vi "NorthWest Window Control_Async.vi"(1 "Desired Window Open %":dbl) -> ()   [LabVIEW 2022 SP3]
uses:
  Anemometry/Anemometry Sub Vis/Globals/Dynamic_call_global.ph.vi
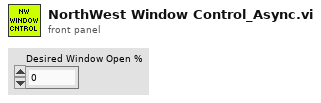
[diagram p1: front panel]
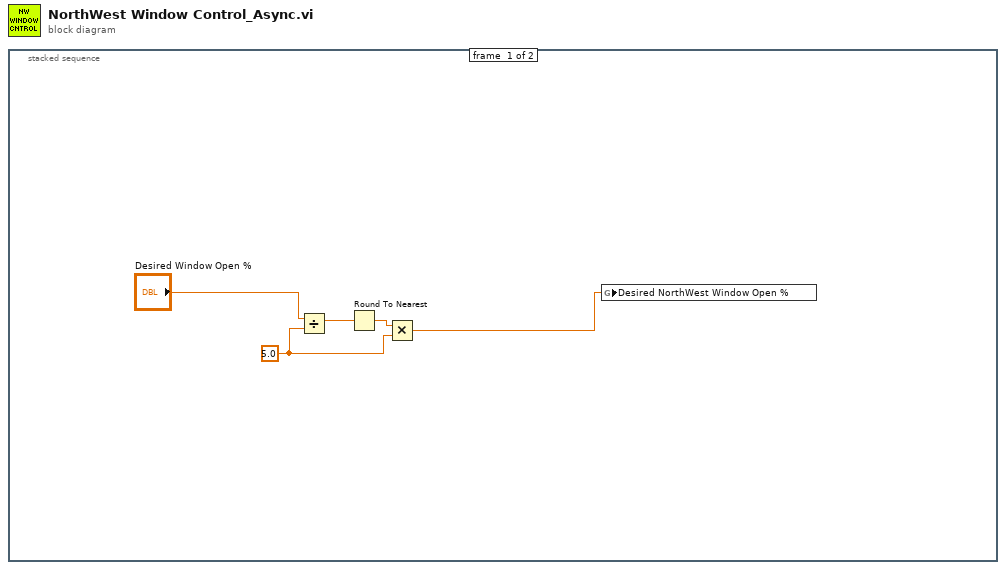
[diagram p0: block diagram]
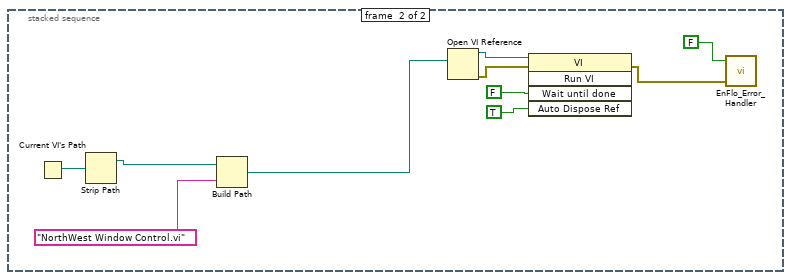
[diagram p2: hidden frame]
diagram:
  n1 = stacked-sequence {
    frame #0 {
      w3 = 5.0 ("y")
      n2 = Divide(x="Desired Window Open %", y=w3) -> (x/y=w5:dbl)
      n3 = Round To Nearest(number=w5) -> (nearest integer value=w4:dbl)
      n4 = Multiply(x=w4, y=w3) -> (x*y=w1:dbl)
      n5 = global write "Dynamic_call_global.ph.vi" "Desired NorthWest Window Open %"(w1) -> ()
    }
    frame #1 {
      n6 = Current VI's Path() -> (path=w11:path)
      n7 = Strip Path(path=w11) -> (stripped path=w10:path)  [unwired: 1 out]
      n8 = Build Path(base path=w10, name or relative path="NorthWest Window Control.vi") -> (appended path=w8:path)
      n9 = Open VI Reference(vi path=w8) -> (vi reference=w13:refnum<vi>, error out=w12:errorcluster)  [unwired: 1 in, 4 out]
      n10 = invoke class="VI" method="Run VI"(reference=w13, error in=w12, "Wait until done"=FALSE, "Auto Dispose Ref"=TRUE) -> (error out=w7:errorcluster)  [unwired: 1 in, 4 out]
      n11 = call "EnFlo_Error_Handler.vi"("error in (no error)"=w7, "Dialog Box (F)"=FALSE ("Dialog Box (T)")) -> ()  [unwired: 2 in, 2 out]
    }
  }
